vi "Populate Database Identifier State machine.vi"() -> ()   [LabVIEW 2013]
uses:
  Controls/Populate databse identifier state.ctl
panel:
  out "State":T1
  out "error out 2":errorcluster
  in  "error out":errorcluster
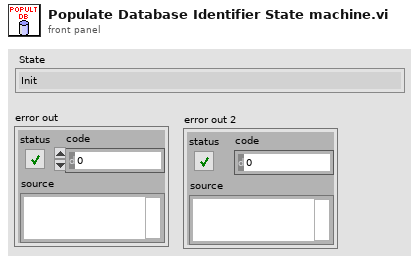
[diagram p1: front panel]
types:
  T1 = typedef "Populate databse identifier state.ctl" = enum16{"Init", "Populate database identifier", "Populate databse devicetype_variable_identifier", "Exit"}
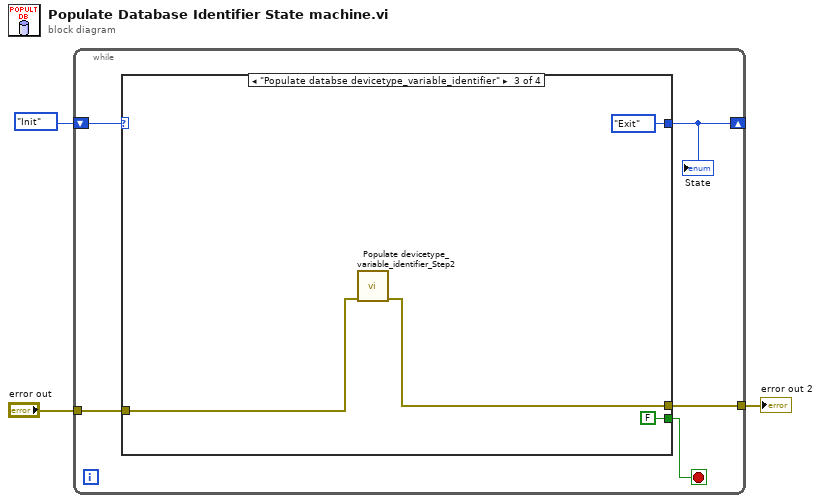
[diagram p0: block diagram]
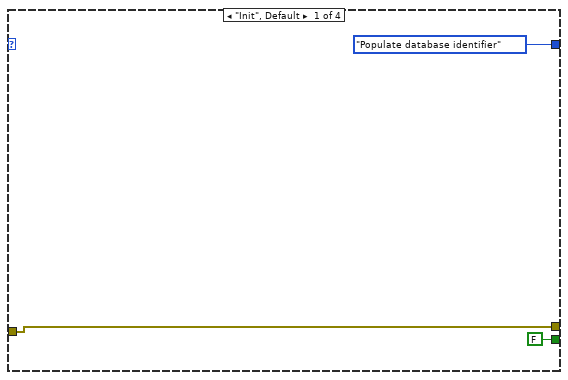
[diagram p2: hidden frame]
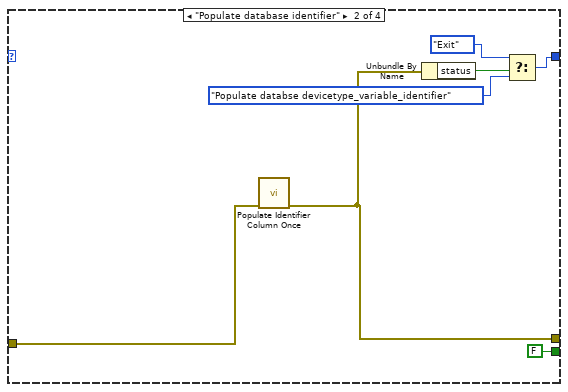
[diagram p3: hidden frame]
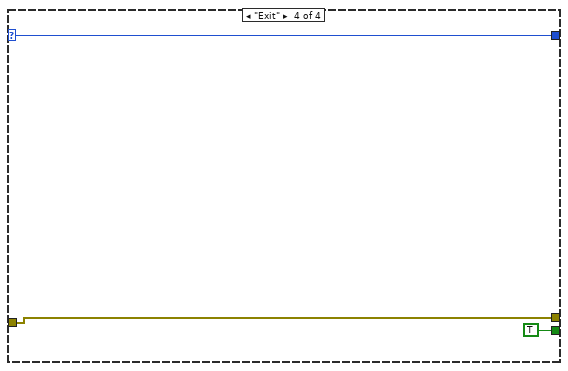
[diagram p4: hidden frame]
diagram:
  n1 = while {
    shift-right: [w7] -> _
    shift-left: Populate_databse_identifier_state."Init" -> [w8]
    tunnel: "error out" -> [w5]
    tunnel: [w4] -> w1
    stop <- w6 stop-if-true
    n2 = case shown="\"Populate databse devicetype_variable_identifier\"" w8 {
      selector: w8 -> [_ _ _ w24]
      tunnel: [Populate_databse_identifier_state."Populate database identifier" w15 Populate_databse_identifier_state."Exit" w24] -> w7
      tunnel: [FALSE FALSE FALSE TRUE] -> w6
      tunnel: w5 -> [w10 w17 w21 w23]
      tunnel: [w10 w16 w20 w23] -> w4
      frame "Init", Default {
      }
      frame "Populate database identifier" {
        n3 = call "Populate Identifier Column Once.vi"("error out"=w17) -> ("error out 2"=w16:errorcluster)  [unwired: 10 in]
        n4 = Unbundle By Name(w16) -> ("status"=w14:bool)
        n5 = Select(t=Populate_databse_identifier_state."Exit", s=w14, f=Populate_databse_identifier_state."Populate databse devicetype_variable_identifier") -> (s? t:f=w15:T1)
      }
      frame "Populate databse devicetype_variable_identifier" {
        n6 = call "Populate devicetype_variable_identifier_Step2.vi"("error out"=w21) -> ("error out 2"=w20:errorcluster)  [unwired: 10 in]
      }
      frame "Exit" {
      }
    }
    "State" <- w7
  }
  "error out 2" <- w1
